vi "ProbePlanAlign.vi"(3 "New Sensor":bool) -> (1 "Accept/Quit":bool)   [LabVIEW 2013]
uses:
  ProbePlanParams.vi
  InstrControl/ProbeStationControl/ProbeStationControl.lvclass
panel:
  in  "Old reference":bool
  in  "Already aligned":bool
  in  "align":bool
  out "Y1 2":i32
  out "X1 2":i32
  in  "Read probeplan reference":bool
  out "Y1280":i32
  out "X1280":i32
  in  "Readtop fiducial":bool
  out "Y1":i32
  out "X1":i32
  in  "Quit":bool
  in  "Accept":bool
  in  "Read bottom fiducial":bool
  # "Map Sensor to ProbePlan"
  # "X"
  # "Y"
  # "First Step:Align the sensor"
  # "as reference for bottom fiducial"
  # "as reference for top fiducial"
  # "Second step: locate the probeplan reference point on the sensor"
  # "as reference for ProbePlan"
  # "X:"
  # "Y:"
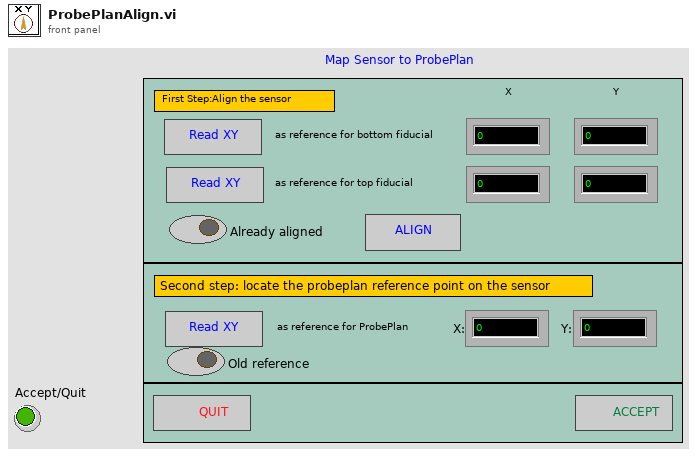
[diagram p1: front panel]
types:
  T1 = cluster{"Strip Number OUT":i32, "X0":i32, "Y0":i32, "X1":i32, "Y1":i32, "Xref":dbl, "Yref":dbl, "ProbePlan type":u32, "Inner pads offset":ext, "Outer pads offset":ext, "l_inner":ext, "l_outer":ext, "strip numbering":u16, "Device Orientation":ext, "Stagger offset":i32, "Yoffset":dbl, "Strip pitch":dbl, "Fiducail separation":dbl, "Radius":ext, "Relative strip angles":dbl, "Probeplan description":string, "ProbePlan array":cluster{"Region":string, "ProbePoints":cluster{"X":dbl, "Y":dbl, "Label":string, "CardViable?":bool}[]}[], "Test ProbePoints":cluster{"Regions Enabled":bool[], "From index":u32[], "To index":u32[]}}
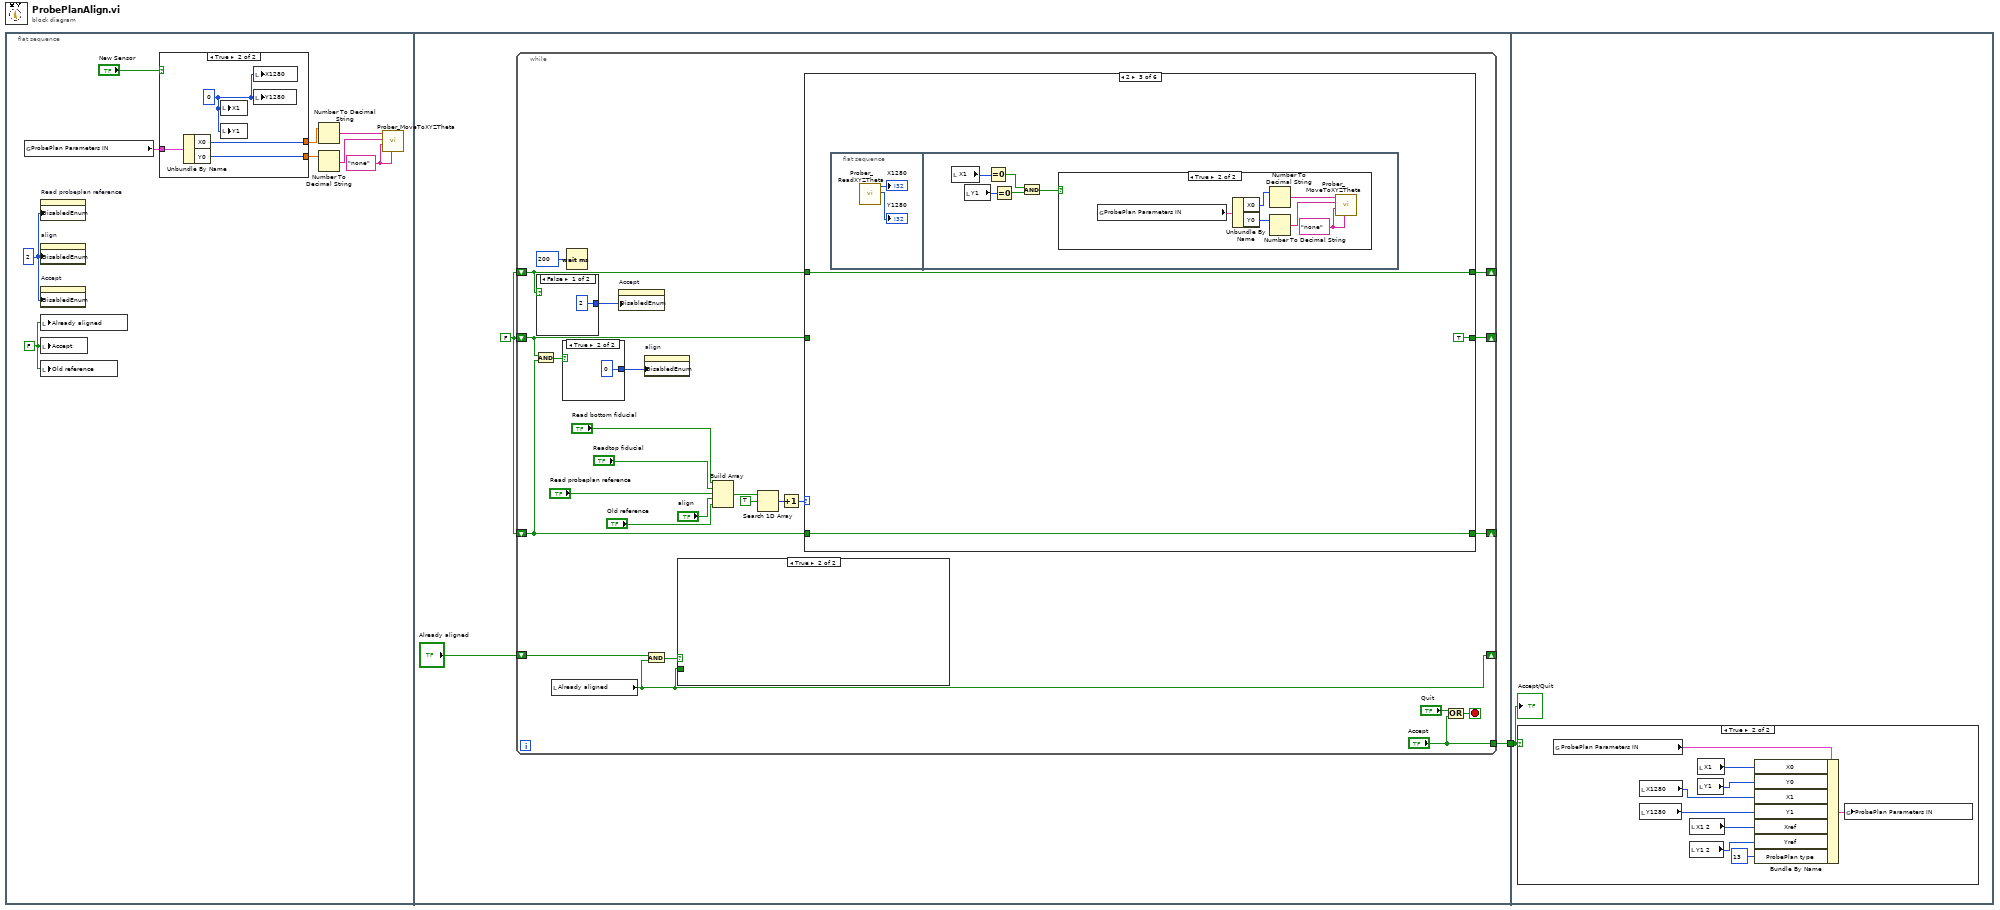
[diagram p0: block diagram]
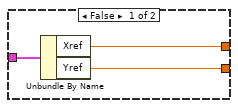
[diagram p2: hidden frame]
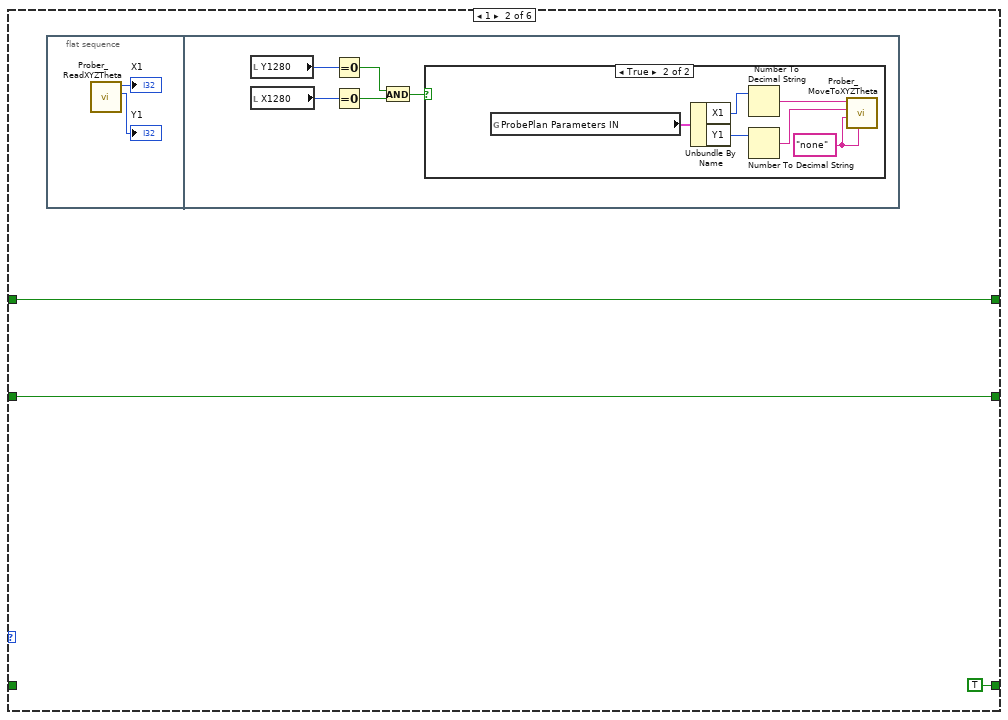
[diagram p4: hidden frame]
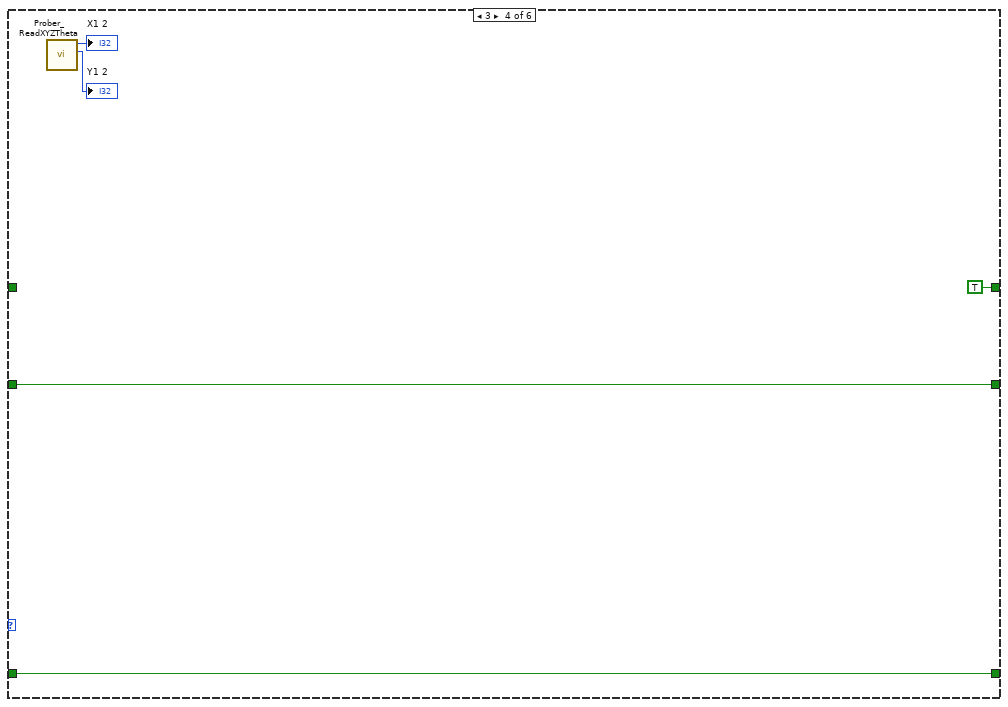
[diagram p7: hidden frame]
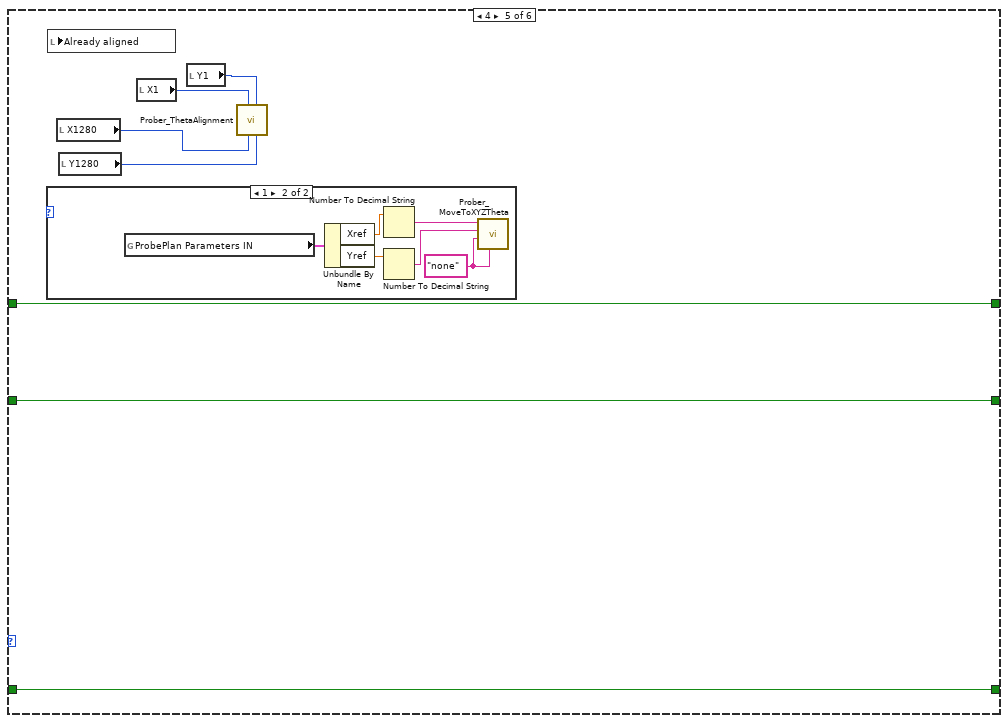
[diagram p8: hidden frame]
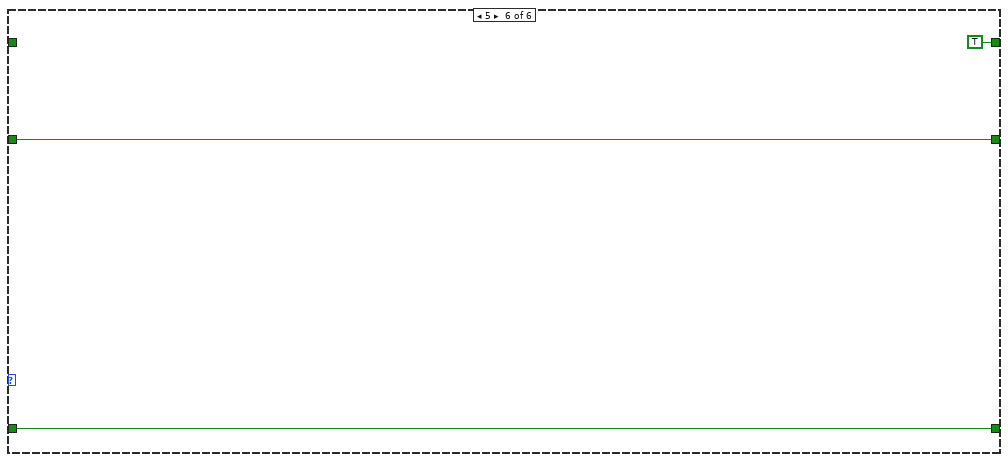
[diagram p10: hidden frame]
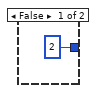
[diagram p11: hidden frame]
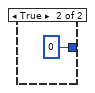
[diagram p12: hidden frame]
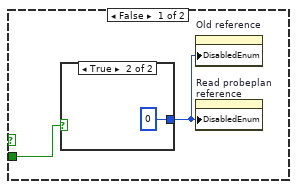
[diagram p13: hidden frame]
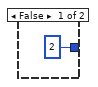
[diagram p14: hidden frame]
diagram:
  n1 = flat-sequence {
    tunnel: [w19] -> w1
    tunnel: w1 -> [w110]
    frame #0 {
      w8 = "none"
      w10 = 2
      w9 = FALSE
      n2 = global read "ProbePlanParams.vi" "ProbePlan Parameters IN"() -> (w4:T1)
      n3 = property on="Read probeplan reference" class="Bool"("DisabledEnum"=w10) -> ()  [unwired: 2 in, 2 out]
      n4 = property on="align" class="Bool"("DisabledEnum"=w10) -> ()  [unwired: 2 in, 2 out]
      n5 = property on="Accept" class="Bool (strict)"("DisabledEnum"=w10) -> ()  [unwired: 2 in, 2 out]
      n6 = local write "Already aligned"(w9) -> ()
      n7 = local write "Accept"(w9) -> ()
      n8 = local write "Old reference"(w9) -> ()
      n9 = case shown="True" "New Sensor" {
        tunnel: w4 -> [w13 w17]
        tunnel: [w12 w16] -> w3
        tunnel: [w11 w15] -> w2
        frame False {
          n10 = Unbundle By Name(w13) -> ("Xref"=w12:dbl, "Yref"=w11:dbl)
        }
        frame True {
          w14 = 0
          n11 = Unbundle By Name(w17) -> ("X0"=w16:i32, "Y0"=w15:i32)
          n12 = local write "X1"(w14) -> ()
          n13 = local write "Y1"(w14) -> ()
          n14 = local write "X1280"(w14) -> ()
          n15 = local write "Y1280"(w14) -> ()
        }
      }
      n16 = Number To Decimal String(number=w3) -> (decimal integer string=w7:string)  [unwired: 1 in]
      n17 = Number To Decimal String(number=w2) -> (decimal integer string=w6:string)  [unwired: 1 in]
      n18 = call-dynamic "Prober_MoveToXYZTheta.vi"("Theta location [mdeg]"=w8, "Z location [µm]"=w8, "Y location [µm]"=w6, "X location [µm]"=w7) -> ()  [unwired: 5 in, 3 out]
    }
    frame #1 {
      w18 = FALSE
      n19 = while {
        shift-right: [w44] -> _
        shift-left: "Already aligned" -> [w27]
        tunnel: ["Accept"] -> w19
        shift-right: [w26] -> _
        shift-left: w18 -> [w29]
        shift-right: [w23] -> _
        shift-left: w18 -> [w24]
        shift-right: [w25] -> _
        shift-left: w18 -> [w28]
        stop <- w42 stop-if-true
        n20 = And(x=w29, y=w28) -> (x .and. y?=w31:bool)
        n21 = case shown="False" w24 {
          tunnel: [2 0] -> w33
          frame False {
          }
          frame True {
          }
        }
        n22 = local read "Already aligned"() -> (w44:bool)
        n23 = case shown="True" w31 {
          tunnel: [2 0] -> w32
          frame False {
          }
          frame True {
          }
        }
        n24 = Wait (ms)(milliseconds to wait=u32 200) -> ()  [unwired: 1 out]
        n25 = property on="Accept" class="Bool (strict)"("DisabledEnum"=w33) -> ()  [unwired: 2 in, 2 out]
        n26 = property on="align" class="Bool"("DisabledEnum"=w32) -> ()  [unwired: 2 in, 2 out]
        n27 = And(x=w27, y=w44) -> (x .and. y?=w45:bool)
        n28 = case shown="True" w45 {
          tunnel: w44 -> [w107 _]
          frame False {
            n29 = case shown="True" w107 {
              tunnel: [2 0] -> w106
              frame False {
              }
              frame True {
              }
            }
            n30 = property on="Old reference" class="Bool (strict)"("DisabledEnum"=w106) -> ()  [unwired: 2 in, 2 out]
            n31 = property on="Read probeplan reference" class="Bool"("DisabledEnum"=w106) -> ()  [unwired: 2 in, 2 out]
          }
          frame True {
          }
        }
        n32 = Build Array("Read bottom fiducial", "Readtop fiducial", "Read probeplan reference", "align", "Old reference") -> (w35:bool[])
        n33 = Search 1D Array(1D array=w35, element=TRUE) -> (index of element=w34:i32)  [unwired: 1 in]
        n34 = Increment(x=w34) -> (x+1=w30:i32)
        n35 = case shown="2" w30 {
          tunnel: w29 -> [w47 w49 _ w82 w87 w100]
          tunnel: w28 -> [w46 _ w67 w81 w88 w99]
          tunnel: [w47 w49 TRUE w82 w87 w100] -> w26
          tunnel: [w46 TRUE w67 w81 w88 w99] -> w25
          tunnel: w24 -> [w48 w51 w65 _ w86 _]
          tunnel: [w48 w51 w65 TRUE w86 TRUE] -> w23
          frame 0, Default {
          }
          frame 1 {
            n36 = flat-sequence {
              frame #0 {
                n37 = call-dynamic "Prober_ReadXYZTheta.vi"() -> ("Y location [µm]"=→"Y1":i32, "X location [µm]"=→"X1":i32)  [unwired: 6 in, 4 out]
              }
              frame #1 {
                n38 = local read "Y1280"() -> (w57:i32)
                n39 = local read "X1280"() -> (w58:i32)
                n40 = Equal To 0?(x=w57) -> (x = 0?=w56:bool)
                n41 = Equal To 0?(x=w58) -> (x = 0?=w55:bool)
                n42 = And(x=w56, y=w55) -> (x .and. y?=w54:bool)
                n43 = case shown="True" w54 {
                  frame False {
                  }
                  frame True {
                    w59 = "none"
                    n44 = global read "ProbePlanParams.vi" "ProbePlan Parameters IN"() -> (w62:T1)
                    n45 = Unbundle By Name(w62) -> ("X1"=w63:i32, "Y1"=w64:i32)
                    n46 = Number To Decimal String(number=w63) -> (decimal integer string=w60:string)  [unwired: 1 in]
                    n47 = Number To Decimal String(number=w64) -> (decimal integer string=w61:string)  [unwired: 1 in]
                    n48 = call-dynamic "Prober_MoveToXYZTheta.vi"("Theta location [mdeg]"=w59, "Z location [µm]"=w59, "Y location [µm]"=w61, "X location [µm]"=w60) -> ()  [unwired: 5 in, 3 out]
                  }
                }
              }
            }
          }
          frame 2 {
            n49 = flat-sequence {
              frame #0 {
                n50 = call-dynamic "Prober_ReadXYZTheta.vi"() -> ("Y location [µm]"=→"Y1280":i32, "X location [µm]"=→"X1280":i32)  [unwired: 6 in, 4 out]
              }
              frame #1 {
                n51 = local read "X1"() -> (w74:i32)
                n52 = local read "Y1"() -> (w73:i32)
                n53 = Equal To 0?(x=w74) -> (x = 0?=w71:bool)
                n54 = Equal To 0?(x=w73) -> (x = 0?=w72:bool)
                n55 = And(x=w71, y=w72) -> (x .and. y?=w70:bool)
                n56 = case shown="True" w70 {
                  frame False {
                  }
                  frame True {
                    w75 = "none"
                    n57 = global read "ProbePlanParams.vi" "ProbePlan Parameters IN"() -> (w78:T1)
                    n58 = Unbundle By Name(w78) -> ("X0"=w79:i32, "Y0"=w80:i32)
                    n59 = Number To Decimal String(number=w79) -> (decimal integer string=w76:string)  [unwired: 1 in]
                    n60 = Number To Decimal String(number=w80) -> (decimal integer string=w77:string)  [unwired: 1 in]
                    n61 = call-dynamic "Prober_MoveToXYZTheta.vi"("Theta location [mdeg]"=w75, "Z location [µm]"=w75, "Y location [µm]"=w77, "X location [µm]"=w76) -> ()  [unwired: 5 in, 3 out]
                  }
                }
              }
            }
          }
          frame 3 {
            n62 = call-dynamic "Prober_ReadXYZTheta.vi"() -> ("Y location [µm]"=→"Y1 2":i32, "X location [µm]"=→"X1 2":i32)  [unwired: 6 in, 4 out]
          }
          frame 4 {
            n63 = case shown="1" {
              selector: _ -> [_ _]
              frame 0, Default {
              }
              frame 1 {
                w93 = "none"
                n64 = global read "ProbePlanParams.vi" "ProbePlan Parameters IN"() -> (w96:T1)
                n65 = Unbundle By Name(w96) -> ("Xref"=w97:dbl, "Yref"=w98:dbl)
                n66 = Number To Decimal String(number=w97) -> (decimal integer string=w94:string)  [unwired: 1 in]
                n67 = Number To Decimal String(number=w98) -> (decimal integer string=w95:string)  [unwired: 1 in]
                n68 = call-dynamic "Prober_MoveToXYZTheta.vi"("Theta location [mdeg]"=w93, "Z location [µm]"=w93, "Y location [µm]"=w95, "X location [µm]"=w94) -> ()  [unwired: 5 in, 3 out]
              }
            }
            n69 = local read "Already aligned"() -> ()  [unwired: 1 in]
            n70 = local read "X1280"() -> (w92:i32)
            n71 = local read "Y1280"() -> (w89:i32)
            n72 = local read "X1"() -> (w91:i32)
            n73 = local read "Y1"() -> (w90:i32)
            n74 = call-dynamic "Prober_ThetaAlignment.vi"("y2"=w89, "y1"=w90, "x2"=w92, "x1"=w91) -> ()  [unwired: 4 in, 4 out]
          }
          frame 5 {
          }
        }
        n75 = Or(x="Quit", y="Accept") -> (x .or. y?=w42:bool)
      }
    }
    frame #2 {
      n76 = case shown="True" w110 {
        frame False {
        }
        frame True {
          n77 = global read "ProbePlanParams.vi" "ProbePlan Parameters IN"() -> (w115:T1)
          n78 = local read "X1280"() -> (w112:i32)
          n79 = local read "Y1280"() -> (w111:i32)
          n80 = local read "X1 2"() -> (w118:i32)
          n81 = local read "Y1 2"() -> (w117:i32)
          n82 = local read "X1"() -> (w114:i32)
          n83 = local read "Y1"() -> (w113:i32)
          n84 = Bundle By Name(cluster=w115, "X0"=w114, "Y0"=w113, "X1"=w112, "Y1"=w111, "Xref"=w118, "Yref"=w117, "ProbePlan type"=13) -> (w119:T1)
          n85 = global write "ProbePlanParams.vi" "ProbePlan Parameters IN"(w119) -> ()
        }
      }
      "Accept/Quit" <- w110
    }
  }
